vi "Open Serial Driver.vi"(0 "port number":u32) -> (1 "input refnum":refnum<visa-resource-name>, 2 "input error":i32, 3 "output refnum":refnum<visa-resource-name>, 4 "output error":i32)   [LabVIEW 2020]
uses:
  serpConfig.vi
panel:
  in  "force re-open":bool
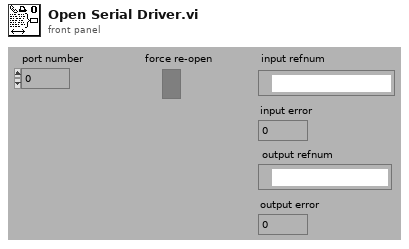
[diagram p1: front panel]
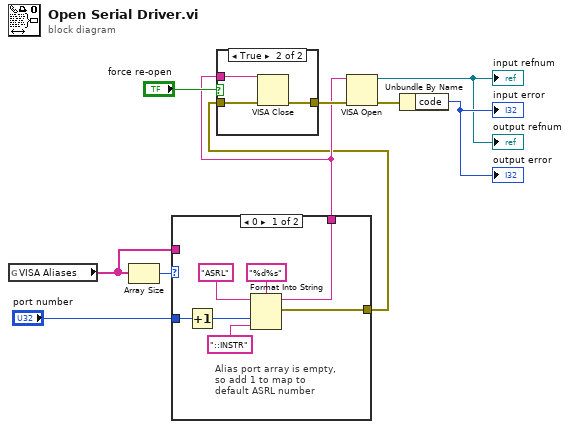
[diagram p0: block diagram]
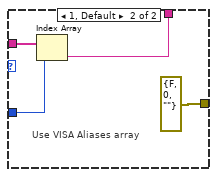
[diagram p2: hidden frame]
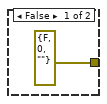
[diagram p3: hidden frame]
diagram:
  n1 = global read "serpConfig.vi" "VISA Aliases"() -> (w4:string[])
  n2 = Array Size(array=w4) -> (size(s)=w5:i32)
  n3 = case shown="0" w5 {
    tunnel: w4 -> [_ w21]
    tunnel: "port number" -> [w17 w20]
    tunnel: [w13 w19] -> w2
    tunnel: [w11 errorcluster {"status"=FALSE, "code"=0, "source"=""} ("error IO")] -> w1
    frame 0 {
      # "Alias port array is empty, so add 1 to map to default ASRL number"
      n4 = Increment(x=w17) -> (x+1=w16:u32)
      n5 = Format Into String(format string="%d%s", initial string="ASRL" ("format string"), w16, "::INSTR" ("format string")) -> (resulting string=w13:string, error out=w11:errorcluster)  [unwired: 1 in]
    }
    frame 1, Default {
      # "Use VISA Aliases array"
      n6 = Index Array(array=w21, index=w20) -> (element=w19:string)
    }
  }
  n7 = case shown="True" "force re-open" {
    tunnel: [errorcluster {"status"=FALSE, "code"=0, "source"=""} ("error out") w25] -> w9
    tunnel: w2 -> [_ w24]
    tunnel: w1 -> [_ w23]
    frame False {
    }
    frame True {
      n8 = VISA Close(VISA resource name=w24, error in (no error)=w23) -> (error out=w25:errorcluster)
    }
  }
  n9 = VISA Open(error in (no error)=w9, VISA resource name=w2) -> (VISA resource name=→"input refnum" →"output refnum":refnum<visa-resource-name>, error out=w8:errorcluster)  [unwired: 3 in]
  n10 = Unbundle By Name(w8) -> ("code"=→"input error" →"output error":i32)
